vi "ReversedEngineering RemoveErrorObjects.vi"(1 "ObjectsIn":refnum<vi>[](array[refnum])) -> (0 "ObjectsOut":refnum<vi>[](array[refnum]))   [LabVIEW 2016]
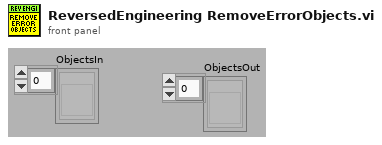
[diagram p1: front panel]
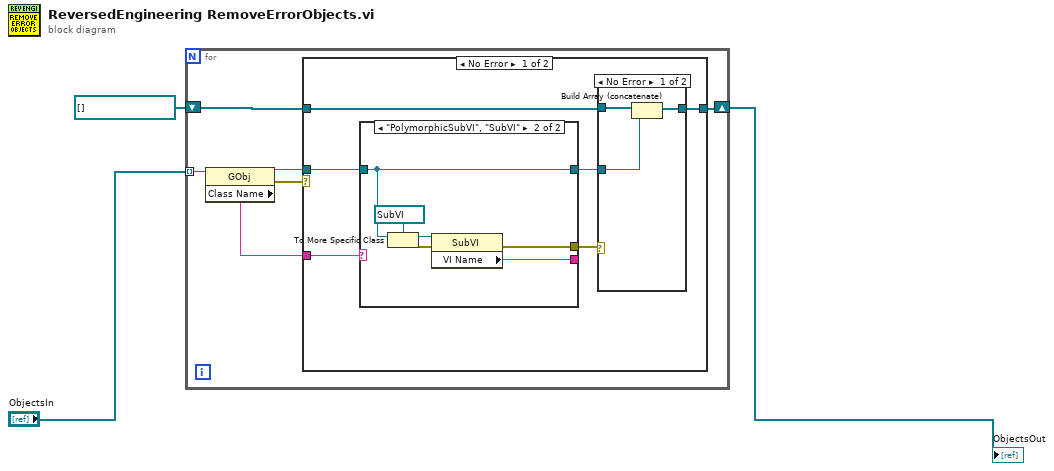
[diagram p0: block diagram]
diagram:
  n1 = for {
    shift-right: [w8] -> w3
    shift-left: refnum<vi>[] [] -> [w9]
    tunnel: "ObjectsIn" -> [w6] mode=indexing
    n2 = property class="GObj"(reference=w6) -> (reference out=w7:refnum<vi>, error out=w5:errorcluster, "Class Name"=w4:string)  [unwired: 1 in]
    n3 = case shown="No Error" w5 {
      tunnel: w9 -> [w15 w27]
      tunnel: [w14 w27] -> w8
      tunnel: w7 -> [w12 _]
      tunnel: w4 -> [w13 _]
      frame No Error {
        n4 = case shown="\"PolymorphicSubVI\", \"SubVI\"" w13 {
          tunnel: w12 -> [w20 w22]
          tunnel: [w20 w22] -> w11
          tunnel: [_ w23] -> w10
          tunnel: [_ w21] -> _
          frame "False", Default {
          }
          frame "PolymorphicSubVI", "SubVI" {
            n5 = To More Specific Class(target class=refnum<vi> refnum ("WhileLoop"), reference=w22) -> (specific class reference=w25:refnum<vi>, error out=w24:errorcluster)  [unwired: 1 in]
            n6 = property class="SubVI"(reference=w25, error in=w24) -> (error out=w23:errorcluster, "VI Name"=w21:string)  [unwired: 1 out]
          }
        }
        n7 = case shown="No Error" w10 {
          tunnel: w15 -> [w18 w19]
          tunnel: [w17 w19] -> w14
          tunnel: w11 -> [w16 _]
          frame No Error {
            n8 = Build Array (concatenate)(w18, w16) -> (w17:refnum<vi>[])
          }
          frame Error {
          }
        }
      }
      frame Error {
      }
    }
  }
  "ObjectsOut" <- w3
